vi "Find Pulse Recorders.vi"(8 "error in (no error)":errorcluster, 9 "Auto launch":bool=TRUE, 10 "Device family":T1(ring), 11 "Monitor-Pulse in":refnum<class "Monitor-Pulse.lvclass">) -> (0 "error out":errorcluster, 1 "Actor names out":string[](array[string]), 2 "Recorders out":refnum<class "Pulse Recorder.lvclass">[](array[class]), 3 "Monitor-Pulse out":refnum<class "Monitor-Pulse.lvclass">)   [LabVIEW 2015, in "Monitor-Pulse.lvclass"]
uses:
  Monitor-Pulse.lvclass
  Measure_core/Pulse Recorders/Pulse Recorder/Pulse Recorder.lvclass
  Measure_core/Pulse Recorders/Pulse Recorder/Pulse Recorder.lvclass/Pulse Recorder.ctl
  Measure_core/Measure Object/Measure Object.lvclass/Measure Object.ctl
  Measure_core/Pulse Recorders/Pulse Recorder/Write Pulse driver.vi
  Measure_core/Measure Object/Write Name.vi
  NHMFL_Core/Libraries/NI-DAQ/DAQmx Digitizer/DAQmx Digitizer.lvclass
  NHMFL_Core/Libraries/NI-DAQ/NI-Scope Digitizer/Ni-Scope Digitizer.lvclass
  NHMFL_Core/Libraries/Red Pitaya/Red Pitaya Digitizer/Red Pitaya Digitizer.lvclass
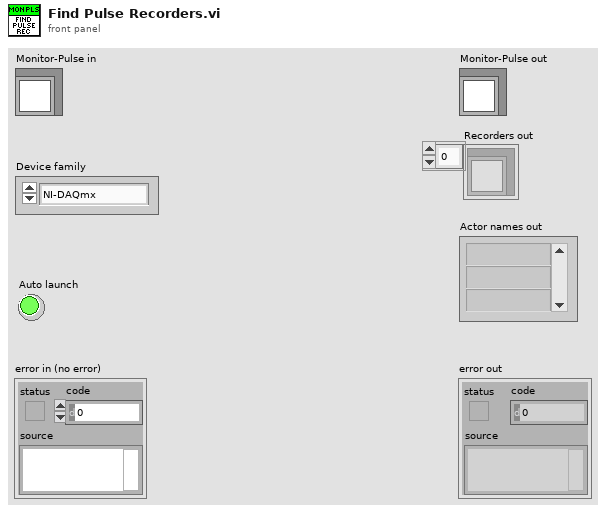
[diagram p1: front panel]
types:
  T1 = enum16{"NI-DAQmx", "NI-Scope", "Red Pitaya", "GaGe"}
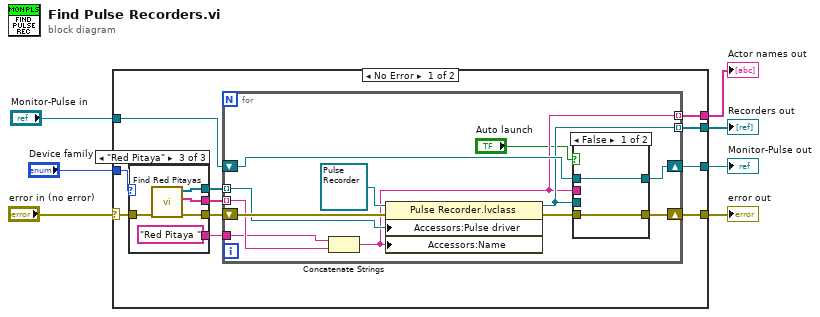
[diagram p0: block diagram]
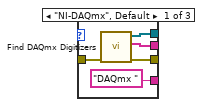
[diagram p2: hidden frame]
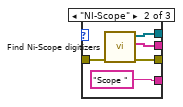
[diagram p3: hidden frame]
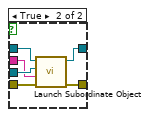
[diagram p4: hidden frame]
diagram:
  n1 = case shown="No Error" "error in (no error)" {
    selector: "error in (no error)" -> [w18 w55]
    tunnel: [w14 w55] -> w6
    tunnel: [w10 w54] -> w4
    tunnel: "Monitor-Pulse in" -> [w11 w54]
    tunnel: [w13 _] -> w3
    tunnel: [w12 _] -> w2
    tunnel: "Device family" -> [w9 _]
    frame No Error {
      n2 = case shown="\"Red Pitaya\"" w9 {
        tunnel: w18 -> [w23 w28 w33]
        tunnel: [w22 w25 w30] -> w17
        tunnel: [w21 w27 w32] -> w16
        tunnel: [w20 w26 w31] -> w15
        tunnel: ["DAQmx " "Scope " "Red Pitaya "] -> w8
        frame "NI-DAQmx", Default {
          n3 = call "Find DAQmx Digitizers.vi"("Error In"=w23) -> ("Error Out"=w21:errorcluster, "Device names"=w20:tag[], "Digitizers out"=w22:refnum<class "Pulse Driver.lvclass">[])  [unwired: 8 in]
        }
        frame "NI-Scope" {
          n4 = call "Find Ni-Scope digitizers.vi"("Error In"=w28) -> ("Error Out"=w27:errorcluster, "Device names out"=w26:string[], "Digitizers out"=w25:refnum<class "Pulse Driver.lvclass">[])  [unwired: 8 in]
        }
        frame "Red Pitaya" {
          n5 = call "Find Red Pitayas.vi"("Error In"=w33) -> ("Error Out"=w32:errorcluster, "Device names"=w31:string[], "Digitizers out"=w30:refnum<class "Pulse Driver.lvclass">[])  [unwired: 7 in, 1 out]
        }
      }
      n6 = for {
        tunnel: w17 -> [w43] mode=indexing
        shift-right: [w37] -> w14
        shift-left: w16 -> [w44]
        tunnel: w15 -> [w42] mode=indexing
        tunnel: [w40] -> w13 mode=indexing
        tunnel: [w36] -> w12 mode=indexing
        shift-right: [w39] -> w10
        shift-left: w11 -> [w41]
        tunnel: w8 -> [w34]
        n7 = Concatenate Strings(w34, w42) -> (w36:string)
        n8 = property class="Pulse Recorder.lvclass"(reference=refnum<class "Pulse Recorder.lvclass"> refnum ("Pulse Recorder.lvclass"), error in=w44, "Accessors:Pulse driver"=w43, "Accessors:Name"=w36) -> (reference out=w40:refnum<class "Pulse Recorder.lvclass">, error out=w38:errorcluster)
        n9 = case shown="False" "Auto launch" {
          tunnel: w41 -> [w47 w53]
          tunnel: w40 -> [_ w52]
          tunnel: [w47 w51] -> w39
          tunnel: w38 -> [w46 w50]
          tunnel: [w46 w49] -> w37
          tunnel: w36 -> [_ w48]
          frame False {
          }
          frame True {
            n10 = call-dynamic "Launch Subordinate Object.vi"("error in (no error)"=w50, "Name"=w48, "Subordinate Object"=w52, "Measure Object in"=w53) -> ("error out"=w49:errorcluster, "Measure Object out"=w51:refnum<class "Monitor-Pulse.lvclass">)  [unwired: 5 in, 1 out]
          }
        }
      }
    }
    frame Error {
    }
  }
  "error out" <- w6
  "Monitor-Pulse out" <- w4
  "Recorders out" <- w3
  "Actor names out" <- w2
